vi "exnSpectralSub move terminal to end of Terminal Data array.vi"(5 "Terminal ID":string, 7 "Terminal Data in":T1[](array[typedef]) {"Terminal Flags" format="%.0b"}) -> (8 "Terminal Data out":T1[](array[typedef]) {"Terminal Flags" format="%.0b"})   [LabVIEW 2020]
uses:
  <vilib>/BlockNodeSupport/TerminalData.ctl
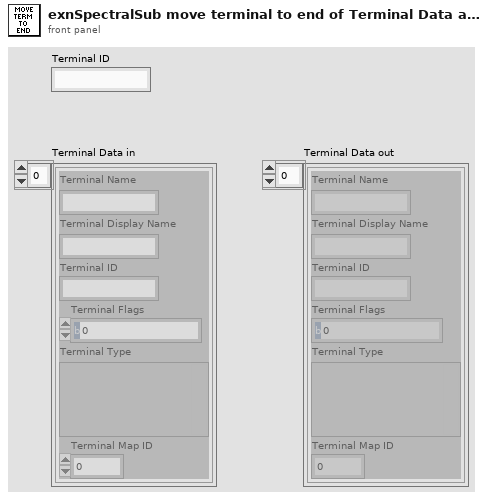
[diagram p1: front panel]
types:
  T1 = typedef "TerminalData.ctl" = cluster{"Terminal Name":string, "Terminal Display Name":string, "Terminal ID":string, "Terminal Flags":i32, "Terminal Type":variant, "Terminal Map ID":i32}
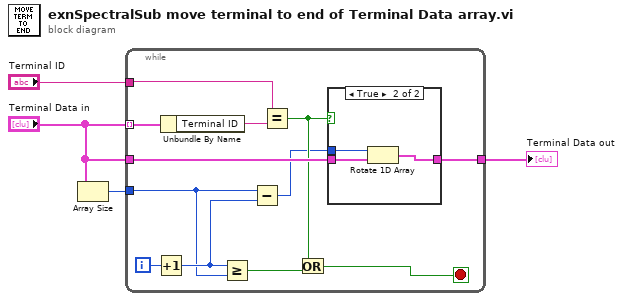
[diagram p0: block diagram]
diagram:
  n1 = Array Size(array="Terminal Data in") -> (size(s)=w3:i32)
  n2 = while {
    tunnel: "Terminal Data in" -> [w16] mode=indexing
    tunnel: "Terminal ID" -> [w14]
    tunnel: w3 -> [w5]
    tunnel: "Terminal Data in" -> [w11]
    tunnel: [w10] -> w1
    i -> [w9]
    stop <- w12 stop-if-true
    n3 = Increment(x=w9) -> (x+1=w6:i32)
    n4 = Unbundle By Name(w16) -> ("Terminal ID"=w15:string)
    n5 = Greater Or Equal?(x=w6, y=w5) -> (x >= y?=w13:bool)
    n6 = Subtract(x=w5, y=w6) -> (x-y=w7:i32)
    n7 = Equal?(x=w14, y=w15) -> (x = y?=w8:bool)
    n8 = Or(x=w8, y=w13) -> (x .or. y?=w12:bool)
    n9 = case shown="True" w8 {
      tunnel: w11 -> [w17 w20]
      tunnel: w7 -> [_ w19]
      tunnel: [w17 w18] -> w10
      frame False {
      }
      frame True {
        n10 = Rotate 1D Array(1:w20, 2:w19) -> (0:w18:T1[])
      }
    }
  }
  "Terminal Data out" <- w1
